vi "Four US Control.vi"(3 "Average Length":i32=10) -> (0 "Distance Front\nRight (A11)":dbl, 1 "Distance Front\nLeft (A13)":dbl, 2 "Instantaneous Distance\nFront Right":dbl, 4 "Instantaneous Distance\nFront Left":dbl)   [LabVIEW 2013]
uses:
  <vilib>/myRIO/Instrument Drivers/Onboard IO/DIO/vis/Smart Open.vi
  <vilib>/myRIO/Instrument Drivers/Onboard IO/DIO/vis/Write.vi
  <vilib>/myRIO/Instrument Drivers/Onboard IO/DIO/vis/Read.vi
  <vilib>/myRIO/Instrument Drivers/Onboard IO/DIO/vis/Open.vi
  <vilib>/myRIO/Common/Instrument Driver Framework/myRIO v1.0/DIO/vis/myRIO v1.1 Open DIO.vi
  <vilib>/myRIO/Common/Instrument Driver Framework/Utilities/vis/Validate Channels.vi
  <vilib>/myRIO/Common/Instrument Driver Framework/myRIO v1.0/DIO/vis/myRIO v1.0 Reserve DIO.vi
  <vilib>/myRIO/Common/Instrument Driver Framework/myRIO v1.0/Resource Manager/vis/myRIO v1.0 Reserve Channel List.vi
  <vilib>/myRIO/Common/Instrument Driver Framework/myRIO v1.0/DIO/vis/myRIO v1.0 Build MUX Configuration DIO.vi
  <vilib>/myRIO/Common/Instrument Driver Framework/myRIO v1.0/Resource Manager/vis/myRIO v1.0 Reserve Channel.vi
  <vilib>/myRIO/Common/Instrument Driver Framework/myRIO v1.0/Resource Manager/vis/myRIO v1.0 Unreserve Channel.vi
  <vilib>/myRIO/Common/Instrument Driver Framework/myRIO v1.0/Resource Manager/vis/myRIO v1.0 Create Configuration List.vi
  <vilib>/myRIO/Common/Instrument Driver Framework/myRIO v1.0/Resource Manager/vis/myRIO v1.0 Build Mutex Name.vi
  <vilib>/myRIO/Common/Instrument Driver Framework/myRIO v1.0/myRIO v1.1 Open.vi
  <vilib>/Utility/VariantDataType/GetNumericInfo.vi
  <vilib>/Utility/error.llb/Error Cluster From Error Code.vi
  <vilib>/myRIO/Common/Instrument Driver Framework/Utilities/vis/IO Manager.vi
  <vilib>/myRIO/Common/Instrument Driver Framework/Utilities/vis/Configuration Manager.vi
  <vilib>/myRIO/Common/Instrument Driver Framework/myRIO v1.0/Resource Manager/vis/myRIO v1.0 Configure IO.vi
  <vilib>/myRIO/Common/Instrument Driver Framework/myRIO v1.0/myRIO v1.0 Close.vi
  <vilib>/myRIO/Common/Instrument Driver Framework/myRIO v1.0/DIO/vis/myRIO v1.0 Write DIO.vi
  <vilib>/myRIO/Common/Instrument Driver Framework/myRIO v1.0/DIO/vis/myRIO v1.0 Read DIO.vi
  <vilib>/ptbypt/NI_PtbyPt.lvlib
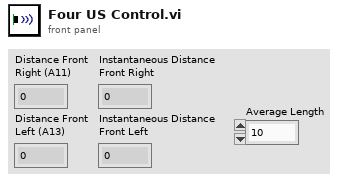
[diagram p1: front panel]
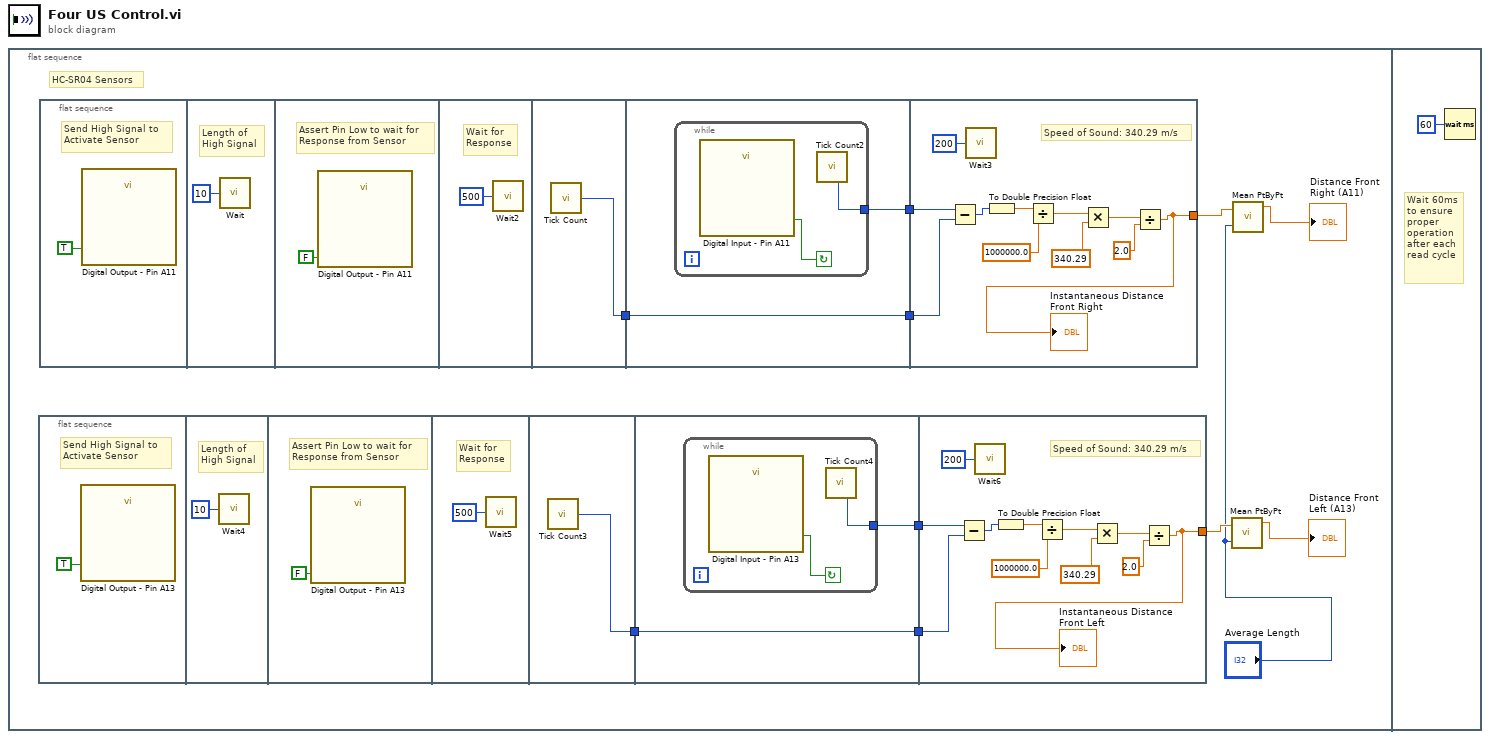
[diagram p0: block diagram]
diagram:
  n1 = flat-sequence {
    frame #0 {
      # "HC-SR04 Sensors"
      n2 = flat-sequence {
        tunnel: [w16] -> w8
        tunnel: [w18] -> w7
        tunnel: [w17] -> w6
        tunnel: w8 -> [w17]
        tunnel: w7 -> [w30]
        tunnel: w6 -> [w29]
        tunnel: [w21] -> w2
        frame #0 {
          # "Send High Signal to \nActivate Sensor"
          n3 = call "Digital Output - Pin A13"("A/DIO2 (Pin 15)"=TRUE ("A/DIO3 (Pin 17)")) -> ()  [unwired: 26 in, 1 out]
        }
        frame #1 {
          # "Length of \nHigh Signal"
          n4 = call "Wait4"("Count(uSec)"=u32 10) -> ()  [unwired: 1 out]
        }
        frame #2 {
          # "Assert Pin Low to wait for\nResponse from Sensor"
          n5 = call "Digital Output - Pin A13"("A/DIO2 (Pin 15)"=FALSE ("A/DIO3 (Pin 17)")) -> ()  [unwired: 26 in, 1 out]
        }
        frame #3 {
          # "Wait for \nResponse"
          n6 = call "Wait5"("Count(uSec)"=u32 500) -> ()  [unwired: 1 out]
        }
        frame #4 {
          n7 = call "Tick Count3"() -> ("Tick Count(uSec)"=w16:u32)
        }
        frame #5 {
          n8 = while {
            tunnel: [w19] -> w18
            stop <- w20 continue-if-true
            n9 = call "Digital Input - Pin A13"() -> ("A/DIO3 (Pin 17)"=w20:bool)  [unwired: 26 in, 1 out]
            n10 = call "Tick Count4"() -> ("Tick Count(uSec)"=w19:u32)
          }
        }
        frame #6 {
          # "Speed of Sound: 340.29 m/s"
          n11 = Subtract(x=w30, y=w29) -> (x-y=w22:u32)
          n12 = call "Wait6"("Count(uSec)"=u32 200) -> ()  [unwired: 1 out]
          n13 = To Double Precision Float(number=w22) -> (double precision float=w23:dbl)
          n14 = Divide(x=w23, y=1000000.0) -> (x/y=w27:dbl)
          n15 = Multiply(x=w27, y=340.29) -> (x*y=w24:dbl)
          n16 = Divide(x=w24, y=2.0) -> (x/y=w21:dbl)
          "Instantaneous Distance\nFront Left" <- w21
        }
      }
      n17 = flat-sequence {
        tunnel: [w36] -> w11
        tunnel: [w37] -> w10
        tunnel: [w38] -> w9
        tunnel: w11 -> [w38]
        tunnel: w10 -> [w50]
        tunnel: w9 -> [w49]
        tunnel: [w41] -> w4
        frame #0 {
          # "Send High Signal to \nActivate Sensor"
          n18 = call "Digital Output - Pin A11"("A/DIO0 (Pin 11)"=TRUE ("A/DIO3 (Pin 17)")) -> ()  [unwired: 26 in, 1 out]
        }
        frame #1 {
          # "Length of \nHigh Signal"
          n19 = call "Wait"("Count(uSec)"=u32 10) -> ()  [unwired: 1 out]
        }
        frame #2 {
          # "Assert Pin Low to wait for\nResponse from Sensor"
          n20 = call "Digital Output - Pin A11"("A/DIO0 (Pin 11)"=FALSE ("A/DIO3 (Pin 17)")) -> ()  [unwired: 26 in, 1 out]
        }
        frame #3 {
          # "Wait for \nResponse"
          n21 = call "Wait2"("Count(uSec)"=u32 500) -> ()  [unwired: 1 out]
        }
        frame #4 {
          n22 = call "Tick Count"() -> ("Tick Count(uSec)"=w36:u32)
        }
        frame #5 {
          n23 = while {
            tunnel: [w39] -> w37
            stop <- w40 continue-if-true
            n24 = call "Digital Input - Pin A11"() -> ("A/DIO1 (Pin 13)"=w40:bool)  [unwired: 26 in, 1 out]
            n25 = call "Tick Count2"() -> ("Tick Count(uSec)"=w39:u32)
          }
        }
        frame #6 {
          # "Speed of Sound: 340.29 m/s"
          n26 = Subtract(x=w50, y=w49) -> (x-y=w42:u32)
          n27 = call "Wait3"("Count(uSec)"=u32 200) -> ()  [unwired: 1 out]
          n28 = To Double Precision Float(number=w42) -> (double precision float=w43:dbl)
          n29 = Divide(x=w43, y=1000000.0) -> (x/y=w47:dbl)
          n30 = Multiply(x=w47, y=340.29) -> (x*y=w44:dbl)
          n31 = Divide(x=w44, y=2.0) -> (x/y=w41:dbl)
          "Instantaneous Distance\nFront Right" <- w41
        }
      }
      n32 = call <vilib>:"Mean PtByPt.vi"("x"=w2, "sample length"="Average Length") -> ("mean"=→"Distance Front\nLeft (A13)":dbl)  [unwired: 2 in, 1 out]
      n33 = call <vilib>:"Mean PtByPt.vi"("x"=w4, "sample length"="Average Length") -> ("mean"=→"Distance Front\nRight (A11)":dbl)  [unwired: 2 in, 1 out]
    }
    frame #1 {
      # "Wait 60ms\nto ensure \nproper \noperation\nafter each \nread cycle"
      n34 = Wait (ms)(milliseconds to wait=u32 60) -> ()  [unwired: 1 out]
    }
  }
